vi "Read Voltage Output .vi"(6 "Settle (1mS)":u32=1, 8 "error in (no error)":errorcluster, 11 "VISA resource name":refnum<visa-resource-name>) -> (0 "error out":errorcluster, 2 "Output Voltage (V)":dbl format="%.4f", 3 "VISA resource name out":refnum<visa-resource-name>)   [LabVIEW 2012, in "TDK-Lambda Z.lvlib"]
doc: "Returns the output voltage measured by the power supply."
uses:
  TDK-Lambda Z.lvlib
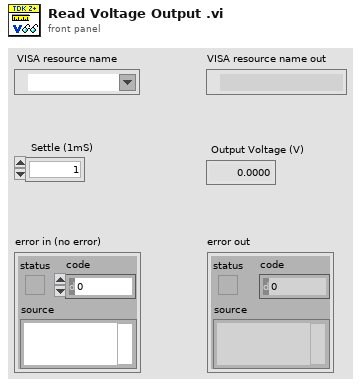
[diagram p1: front panel]
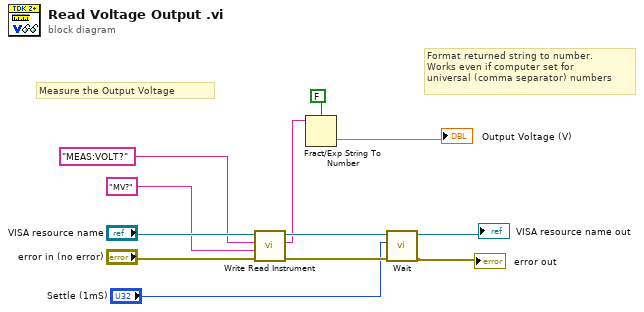
[diagram p0: block diagram]
diagram:
  # "Format returned string to number.\nWorks even if computer set for \nuniversal (comma separator) numbers"
  # "Measure the Output Voltage"
  n1 = call "Write Read Instrument.vi"("error in (no error)"="error in (no error)", "GEN  Write Command/Query"="MV?" ("format string"), "SCPI  Write Command/Query"="MEAS:VOLT?" ("format string"), "VISA resource name"="VISA resource name") -> ("error out"=w9:errorcluster, "Response"=w1:string, "VISA resource name out"=w10:refnum<visa-resource-name>)  [unwired: 5 in]
  n2 = Fract/Exp String To Number(use system decimal point (T)=FALSE, string=w1) -> (number=→"Output Voltage (V)":dbl)  [unwired: 2 in, 1 out]
  n3 = call "Wait.vi"("error in (no error)"=w9, "Wait (1mS)"="Settle (1mS)", "VISA resource name"=w10) -> ("error out"=→"error out":errorcluster, "VISA resource name out"=→"VISA resource name out":refnum<visa-resource-name>)  [unwired: 7 in]
